vi "configuracion-manual-lentes-funciona.vi"() -> ()   [LabVIEW 2024]
uses:
  TG JD - running/TG Juan Diego/Documentos de Labview/160620 Optotune Lens Driver 4 Labview package/Hello Optotune Lens (30.06.2015)/Calibration.ctl
  <vilib>/Instr/_visa.llb/VISA Configure Serial Port (Instr).vi
panel:
  out "error out 4":errorcluster
  out "error out 3":errorcluster
  out "DPT INICIALES D":dbl
  in  "Potencia inicial lente derecho":dbl(slide) scale=-3.0..3.0
  in  "error in (no error) 3":errorcluster
  in  "error in (no error) 4":errorcluster
  out "DPT INICIALES I":dbl
  in  "Potencia inicial lente izquierdo":dbl(slide) scale=-3.0..3.0
  in  "VISA resource name 2":string="COM10"
  out "VISA resource name out 2":string
  out "Command to Port":string
  out "Data":string
  out "OK":bool
  out "Calibration 2":T1 {"Max Current A" format="%#_g mA"; "Max Current B" format="%#_g mA"; "UCL A" format="%#_g mA"; "LCL A" format="%#_g mA"; "UCL B" format="%#_g mA"; "LCL B" format="%#_g mA"}
  out "VISA resource name out":string
  out "ID":u16
  in  "Calibration":T1={"Max Current A"=293.0, "Max Current B"=293.0, "UCL A"=300.0, "UCL B"=300.0, "LCL A"=0.0, "LCL B"=0.0} {"Max Current A" format="%#_g mA"; "Max Current B" format="%#_g mA"; "UCL A" format="%#_g mA"; "LCL A" format="%#_g mA"; "UCL B" format="%#_g mA"; "LCL B" format="%#_g mA"}
  in  "VISA resource name":string="COM11"
  in  "Parar adquisicion":bool
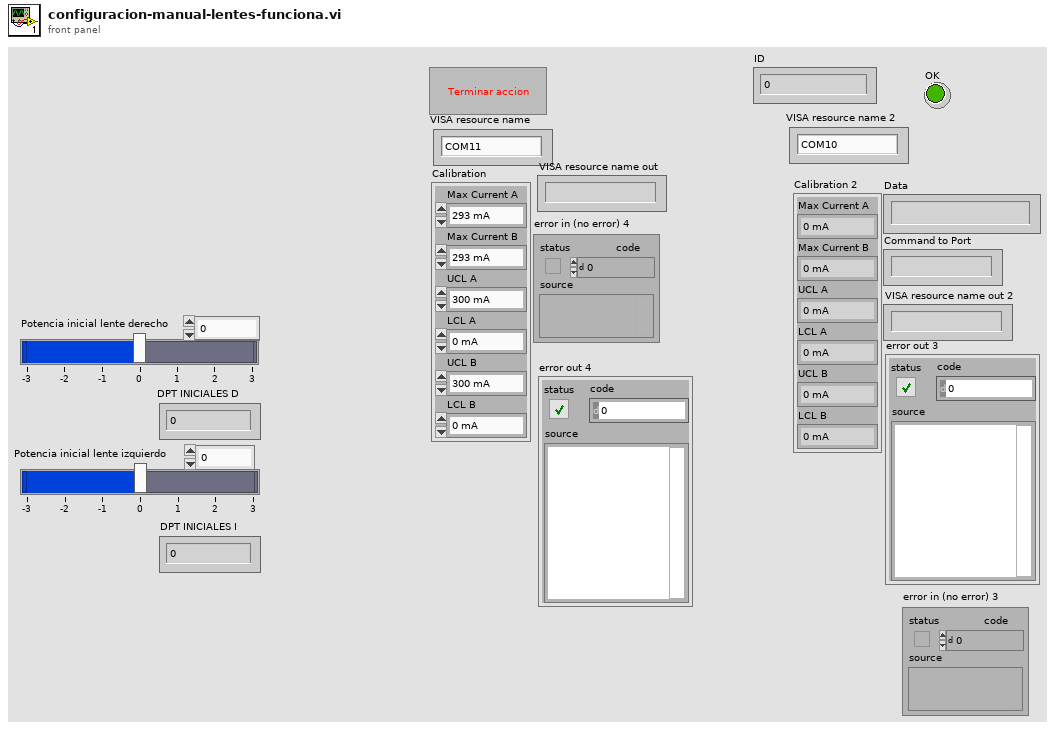
[diagram p1: front panel]
types:
  T1 = typedef "Calibration.ctl" = cluster{"Max Current A":dbl, "Max Current B":dbl, "UCL A":dbl, "UCL B":dbl, "LCL A":dbl, "LCL B":dbl}
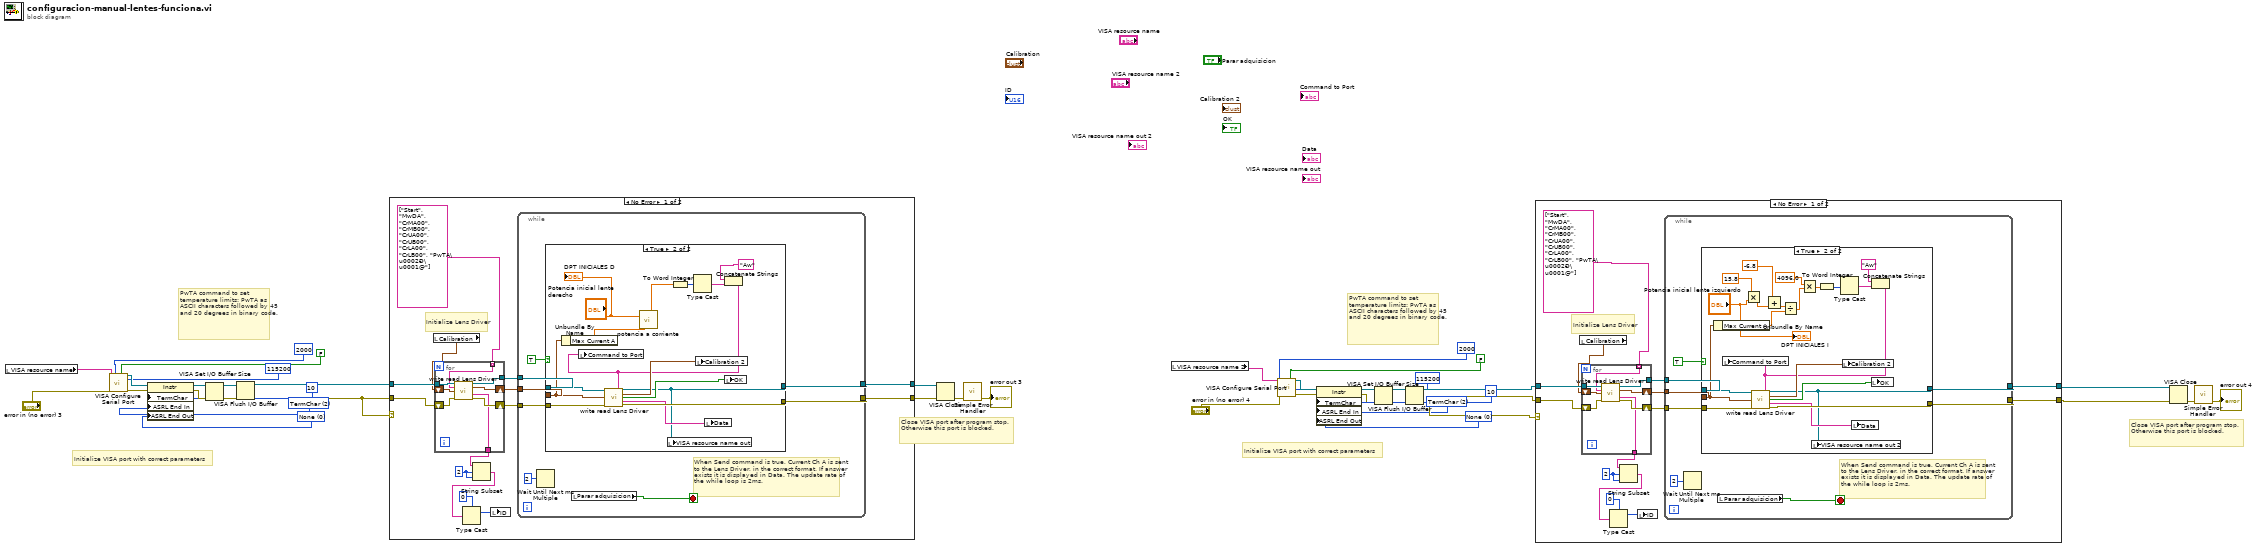
[diagram p0: block diagram]
diagram:
  w21 = u16 0 items=["None", "Last Bit", "TermChar", "Break"] ("Serial Settings:End Mode for Writes")
  w20 = u16 2 items=["None", "Last Bit", "TermChar"] ("Serial Settings:End Mode for Reads")
  w34 = u16 0 items=["None", "Last Bit", "TermChar", "Break"] ("Serial Settings:End Mode for Writes")
  w33 = u16 2 items=["None", "Last Bit", "TermChar"] ("Serial Settings:End Mode for Reads")
  # "Close VISA port after program stop. Otherwise this port is blocked."
  # "Close VISA port after program stop. Otherwise this port is blocked."
  # "PwTA command to set temperature limits: PwTA as ASCII characters followed by 45 and 20 degrees in binary code."
  # "Initialize VISA port with correct parameters"
  # "PwTA command to set temperature limits: PwTA as ASCII characters followed by 45 and 20 degrees in binary code."
  # "Initialize VISA port with correct parameters"
  n1 = local read "VISA resource name"() -> (w11:string)
  n2 = call-poly "VISA Configure Serial Port"("VISA resource name"=w11, "timeout (10sec)"=u32 2000, "Enable Termination\nChar (T)"=FALSE ("Enable Termination\nChar (T)"), "baud rate (9600)"=u32 115200, "error in (no error)"="error in (no error) 3") -> ("VISA resource name out"=w16:refnum<visa-resource-name>, "error out"=w18:errorcluster)  [unwired: 9 in]
  n3 = property class="Instr"(reference=w16, error in=w18, "TermChar"=u8 10 ("Message Based Settings:Termination Character"), "ASRL End In"=w20, "ASRL End Out"=w21) -> (reference out=w17:refnum<visa-resource-name>, error out=w19:errorcluster)
  n4 = VISA Set I/O Buffer Size(VISA resource name=w17, error in (no error)=w19) -> (VISA resource name out=w23:refnum<visa-resource-name>, error out=w24:errorcluster)  [unwired: 2 in]
  n5 = VISA Flush I/O Buffer(VISA resource name=w23, error in (no error)=w24) -> (VISA resource name out=w10:refnum<visa-resource-name>, error out=w9:errorcluster)  [unwired: 1 in]
  n6 = case shown="No Error" w9 {
    tunnel: w9 -> [w54 w88]
    tunnel: w10 -> [w53 w89]
    tunnel: [w52 w88] -> w5
    tunnel: [w51 w89] -> w6
    frame No Error {
      w50 = 2 ("length (rest)")
      # "Initialize Lens Driver"
      n7 = local read "Calibration"() -> (w42:T1)
      n8 = for {
        tunnel: w53 -> [w86]
        tunnel: [w83] -> w45
        tunnel: string[] ["Start", "MwDA", "CrMA00", "CrMB00", "CrUA00", "CrUB00", "CrLA00", "CrLB00", "PwTA\u0002Ð\u0001@"] -> [w81] mode=indexing
        tunnel: [w80] -> w44
        shift-right: [w84] -> w46
        shift-left: w42 -> [w85]
        shift-right: [w82] -> w47
        shift-left: w54 -> [w87]
        n9 = call "write read Lens Driver.vi"("VISA resource name"=w86, "command"=w81, "Calibration"=w85, "error in (no error)"=w87) -> ("VISA resource name out"=w83:refnum<visa-resource-name>, "Calibration 2"=w84:T1, "Data"=w80:string, "error out"=w82:errorcluster)  [unwired: 4 in, 4 out]
      }
      n10 = String Subset(string=w44, offset (0)=w50, length (rest)=w50) -> (substring=w48:string)
      n11 = Type Cast(type=u16 0 ("length (rest)"), x=w48) -> (*(type *) &x=w43:u16)
      n12 = local write "ID"(w43) -> ()
      n13 = while {
        tunnel: [w56] -> w52
        tunnel: [w57] -> w51
        tunnel: w47 -> [w62]
        tunnel: w46 -> [w61]
        tunnel: w45 -> [w60]
        stop <- w55 stop-if-true
        # "When Send command is true, Current Ch A is sent to the Lens Driver, in the correct format. If answer exists it is displayed in Data. The update rate of the while loop is 2ms."
        n14 = Wait Until Next ms Multiple(millisecond multiple=u32 2) -> ()  [unwired: 1 out]
        n15 = case shown="True" TRUE ("Send command") {
          tunnel: [w64 w79] -> w56
          tunnel: w62 -> [w64 w78]
          tunnel: w61 -> [_ w69]
          tunnel: w60 -> [w63 w77]
          tunnel: [w63 w70] -> w57
          frame False {
          }
          frame True {
            n16 = Unbundle By Name(w69) -> ("Max Current A"=w68:dbl)
            n17 = call "potencia a corriente.vi"("Max current A"=w68, "Potencia"="Potencia inicial lente derecho") -> ("Corriente"=w66:dbl)
            n18 = To Word Integer(number=w66) -> (16bit integer=w76:i16)
            n19 = Type Cast(x=w76) -> (*(type *) &x=w75:string)  [unwired: 1 in]
            n20 = Concatenate Strings("Aw", w75) -> (w72:string)
            n21 = local write "Command to Port"(w72) -> ()
            n22 = call "write read Lens Driver.vi"("VISA resource name"=w77, "command"=w72, "Calibration"=w69, "error in (no error)"=w78) -> ("VISA resource name out"=w70:refnum<visa-resource-name>, "Calibration 2"=w74:T1, "OK"=w73:bool, "Data"=w71:string, "error out"=w79:errorcluster)  [unwired: 4 in, 3 out]
            n23 = local write "VISA resource name out"(w70) -> ()
            n24 = local write "Calibration 2"(w74) -> ()
            n25 = local write "Data"(w71) -> ()
            n26 = local write "OK"(w73) -> ()
            "DPT INICIALES D" <- "Potencia inicial lente derecho"
          }
        }
        n27 = local read "Parar adquisicion"() -> (w55:bool)
      }
    }
    frame Error {
    }
  }
  n28 = VISA Close(VISA resource name=w6, error in (no error)=w5) -> (error out=w8:errorcluster)
  n29 = call <vilib>:"Simple Error Handler.vi"("error in (no error)"=w8) -> ("error out"=→"error out 3":errorcluster)  [unwired: 4 in, 4 out]
  n30 = local read "VISA resource name 2"() -> (w25:string)
  n31 = call-poly "VISA Configure Serial Port"("VISA resource name"=w25, "timeout (10sec)"=u32 2000, "Enable Termination\nChar (T)"=FALSE ("Enable Termination\nChar (T)"), "baud rate (9600)"=u32 115200, "error in (no error)"="error in (no error) 4") -> ("VISA resource name out"=w29:refnum<visa-resource-name>, "error out"=w31:errorcluster)  [unwired: 9 in]
  n32 = property class="Instr"(reference=w29, error in=w31, "TermChar"=u8 10 ("Message Based Settings:Termination Character"), "ASRL End In"=w33, "ASRL End Out"=w34) -> (reference out=w30:refnum<visa-resource-name>, error out=w32:errorcluster)
  n33 = VISA Set I/O Buffer Size(VISA resource name=w30, error in (no error)=w32) -> (VISA resource name out=w36:refnum<visa-resource-name>, error out=w37:errorcluster)  [unwired: 2 in]
  n34 = VISA Flush I/O Buffer(VISA resource name=w36, error in (no error)=w37) -> (VISA resource name out=w39:refnum<visa-resource-name>, error out=w38:errorcluster)  [unwired: 1 in]
  n35 = case shown="No Error" w38 {
    tunnel: w38 -> [w103 w143]
    tunnel: w39 -> [w102 w144]
    tunnel: [w101 w143] -> w2
    tunnel: [w100 w144] -> w1
    frame No Error {
      w99 = 2 ("length (rest)")
      # "Initialize Lens Driver"
      n36 = local read "Calibration"() -> (w91:T1)
      n37 = for {
        tunnel: w102 -> [w141]
        tunnel: [w138] -> w94
        tunnel: string[] ["Start", "MwDA", "CrMA00", "CrMB00", "CrUA00", "CrUB00", "CrLA00", "CrLB00", "PwTA\u0002Ð\u0001@"] -> [w136] mode=indexing
        tunnel: [w135] -> w93
        shift-right: [w139] -> w95
        shift-left: w91 -> [w140]
        shift-right: [w137] -> w96
        shift-left: w103 -> [w142]
        n38 = call "write read Lens Driver.vi"("VISA resource name"=w141, "command"=w136, "Calibration"=w140, "error in (no error)"=w142) -> ("VISA resource name out"=w138:refnum<visa-resource-name>, "Calibration 2"=w139:T1, "Data"=w135:string, "error out"=w137:errorcluster)  [unwired: 4 in, 4 out]
      }
      n39 = String Subset(string=w93, offset (0)=w99, length (rest)=w99) -> (substring=w97:string)
      n40 = Type Cast(type=u16 0 ("length (rest)"), x=w97) -> (*(type *) &x=w92:u16)
      n41 = local write "ID"(w92) -> ()
      n42 = while {
        tunnel: [w105] -> w101
        tunnel: [w106] -> w100
        tunnel: w96 -> [w111]
        tunnel: w95 -> [w110]
        tunnel: w94 -> [w109]
        stop <- w104 stop-if-true
        # "When Send command is true, Current Ch A is sent to the Lens Driver, in the correct format. If answer exists it is displayed in Data. The update rate of the while loop is 2ms."
        n43 = Wait Until Next ms Multiple(millisecond multiple=u32 2) -> ()  [unwired: 1 out]
        n44 = case shown="True" TRUE ("Send command") {
          tunnel: [w113 w134] -> w105
          tunnel: w111 -> [w113 w133]
          tunnel: w110 -> [_ w121]
          tunnel: w109 -> [w112 w132]
          tunnel: [w112 w122] -> w106
          frame False {
          }
          frame True {
            n45 = Unbundle By Name(w121) -> ("Max Current A"=w120:dbl)
            n46 = Multiply(x=15.8, y="Potencia inicial lente izquierdo") -> (x*y=w118:dbl)
            n47 = Add(x=-6.8, y=w118) -> (x+y=w116:dbl)
            n48 = Divide(x=w116, y=w120) -> (x/y=w119:dbl)
            n49 = Multiply(x=4096.0, y=w119) -> (x*y=w130:dbl)
            n50 = To Word Integer(number=w130) -> (16bit integer=w129:i16)
            n51 = Type Cast(x=w129) -> (*(type *) &x=w128:string)  [unwired: 1 in]
            n52 = Concatenate Strings("Aw", w128) -> (w124:string)
            n53 = local write "Command to Port"(w124) -> ()
            n54 = call "write read Lens Driver.vi"("VISA resource name"=w132, "command"=w124, "Calibration"=w121, "error in (no error)"=w133) -> ("VISA resource name out"=w122:refnum<visa-resource-name>, "Calibration 2"=w126:T1, "OK"=w125:bool, "Data"=w123:string, "error out"=w134:errorcluster)  [unwired: 4 in, 3 out]
            n55 = local write "VISA resource name out 2"(w122) -> ()
            n56 = local write "Calibration 2"(w126) -> ()
            n57 = local write "Data"(w123) -> ()
            n58 = local write "OK"(w125) -> ()
            "DPT INICIALES I" <- "Potencia inicial lente izquierdo"
          }
        }
        n59 = local read "Parar adquisicion"() -> (w104:bool)
      }
    }
    frame Error {
    }
  }
  n60 = VISA Close(VISA resource name=w1, error in (no error)=w2) -> (error out=w4:errorcluster)
  n61 = call <vilib>:"Simple Error Handler.vi"("error in (no error)"=w4) -> ("error out"=→"error out 4":errorcluster)  [unwired: 4 in, 4 out]
